vi "FormatTree&TableStyle.vi"(7 "Format Command":T1, 8 "Error In":errorcluster, 9 "Row Index":i32, 10 "Array of Table references":refnum<vi>[](array[refnum]), 11 "Array of Tree references":refnum<vi>[](array[refnum])) -> (0 "Error Out":errorcluster)   [LabVIEW 2012]
doc: "SciScan 1.2 160622\nThis VI implements the formatting of table data which includes highlighting, unhighlighting, and modifying visible rows (due to scrolling).\n\n<b>INPUTS</b>\n--------\n<b>Format Command </b> - Formatting action needs to be be taken\n<b>Table references array </b>- Array containing references of the tables of interest\n<b>Row </b>- Row number that needs to be fromatted"
uses:
  FormatTree&TableStyle_Commands.ctl
  <vilib>/Utility/miscctls.llb/LVRowAndColumnTypeDef.ctl
  <vilib>/Utility/miscctls.llb/LVNodeAndColumnTypeDef.ctl
  <vilib>/Utility/miscctls.llb/LVRowAndColumnUnsignedTypeDef.ctl
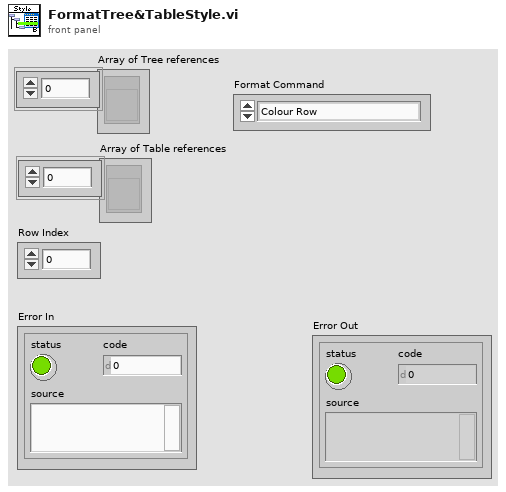
[diagram p1: front panel]
types:
  T1 = typedef "FormatTree&TableStyle_Commands.ctl" = enum16{"Colour Row", "Uncolour Row", "Bold Row", "Unbold Row", "Clear", "UpdateVisibleRows"}
  T2 = typedef "LVRowAndColumnTypeDef.ctl" = cluster{"Row":i32, "Column":i32}
  T3 = typedef "LVRowAndColumnUnsignedTypeDef.ctl" = cluster{"Row":u32, "Column":u32}
  T4 = typedef "LVNodeAndColumnTypeDef.ctl" = cluster{"Node":string, "Column":i32}
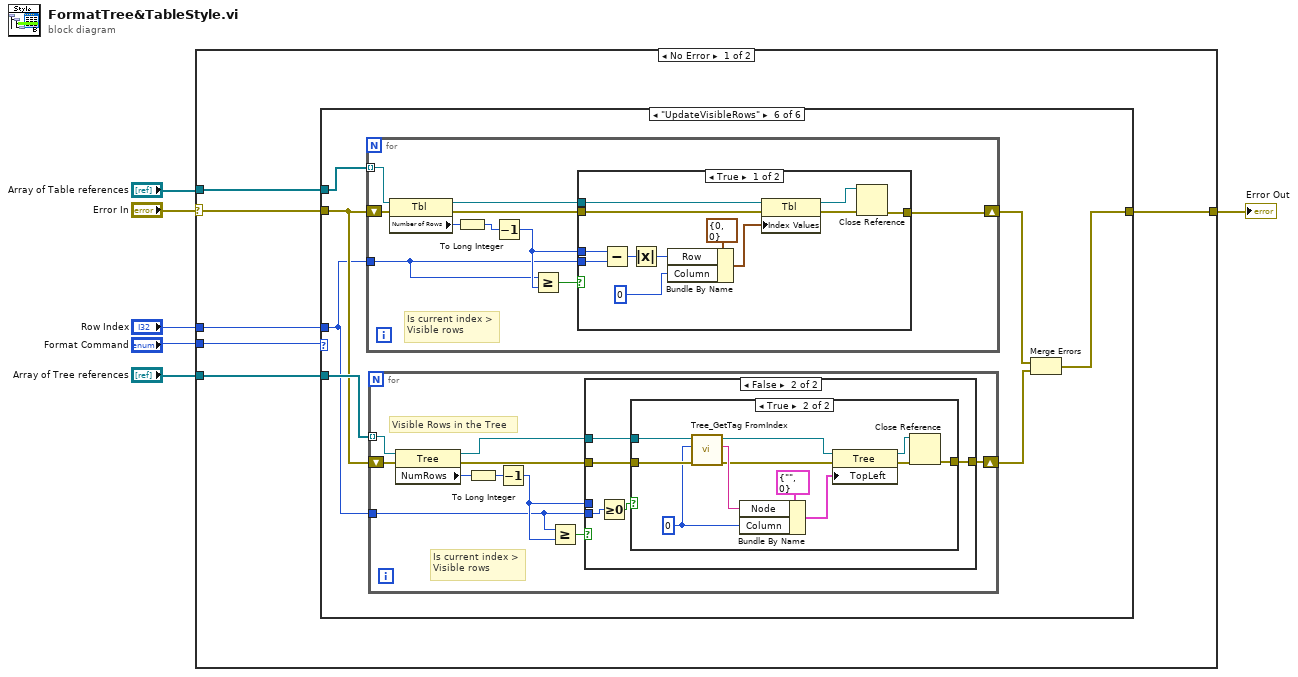
[diagram p0: block diagram]
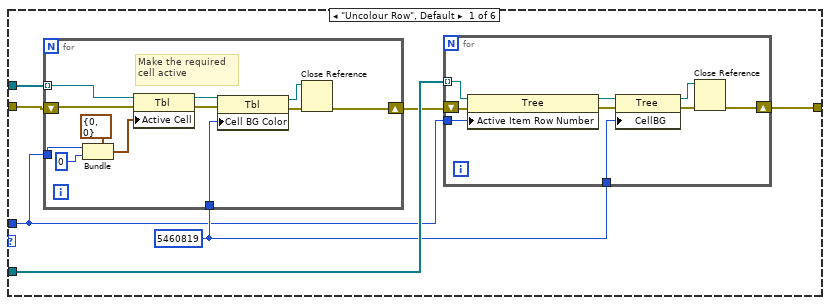
[diagram p2: hidden frame]
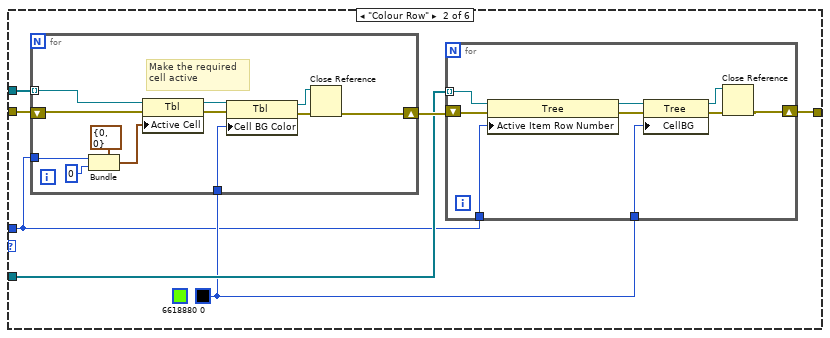
[diagram p3: hidden frame]
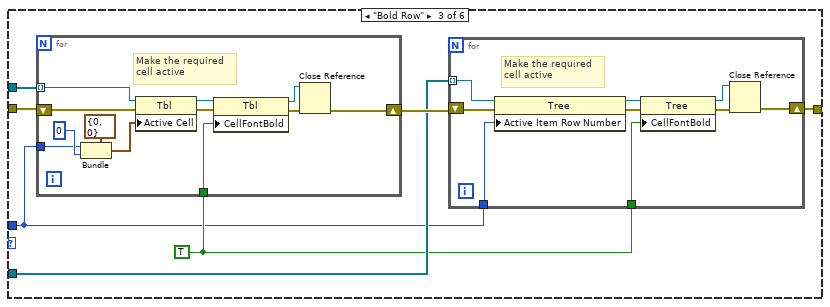
[diagram p4: hidden frame]
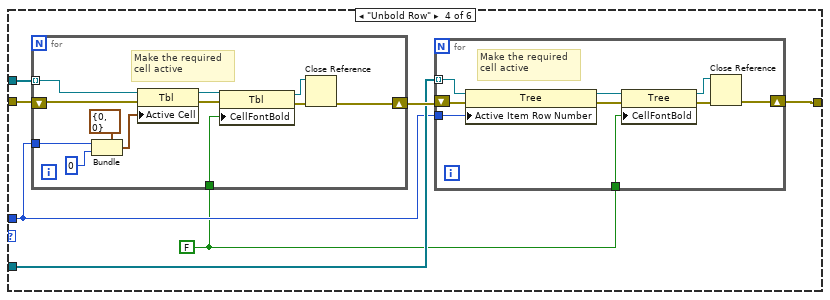
[diagram p5: hidden frame]
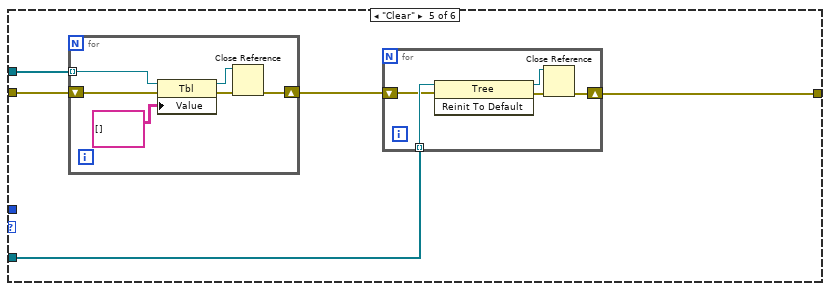
[diagram p6: hidden frame]
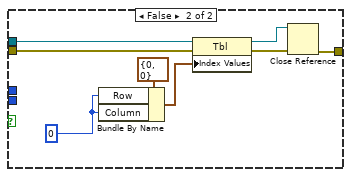
[diagram p7: hidden frame]
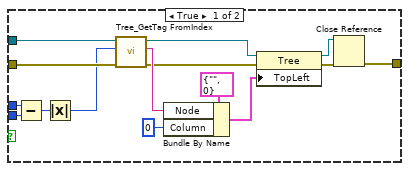
[diagram p8: hidden frame]
diagram:
  n1 = case shown="No Error" "Error In" {
    selector: "Error In" -> [w12 w220]
    tunnel: "Row Index" -> [w10 _]
    tunnel: [w9 w220] -> w4
    tunnel: "Array of Table references" -> [w11 _]
    tunnel: "Format Command" -> [w8 _]
    tunnel: "Array of Tree references" -> [w7 _]
    frame No Error {
      n2 = case shown="\"UpdateVisibleRows\"" w8 {
        tunnel: w12 -> [w19 w46 w74 w102 w128 w145]
        tunnel: w11 -> [w18 w45 w73 w101 w129 w146]
        tunnel: w10 -> [w13 w41 w69 w99 _ w144]
        tunnel: [w15 w43 w71 w98 w125 w141] -> w9
        tunnel: w7 -> [w17 w44 w72 w100 w127 w147]
        frame "Uncolour Row", Default {
          w14 = u32 5460819 ("Active Cell:Cell Background Color")
          n3 = for {
            tunnel: w18 -> [w26] mode=indexing
            tunnel: w14 -> [w24]
            shift-right: [w25] -> w16
            shift-left: w19 -> [w27]
            tunnel: w13 -> [w20]
            # "Make the required cell active"
            n4 = Bundle(cluster=T2 {"Row"=0, "Column"=0} ("Active Cell:Active Cell"), "Row"=w20, "Column"=0) -> (w22:T2)
            n5 = property class="Tbl"(reference=w26, error in=w27, "Active Cell"=w22) -> (reference out=w31:refnum<vi>, error out=w30:errorcluster)
            n6 = property class="Tbl"(reference=w31, error in=w30, "Cell BG Color"=w24) -> (reference out=w28:refnum<vi>, error out=w29:errorcluster)
            n7 = Close Reference(reference=w28, error in (no error)=w29) -> (error out=w25:errorcluster)
          }
          n8 = for {
            tunnel: w17 -> [w40] mode=indexing
            tunnel: w13 -> [w39]
            tunnel: w14 -> [w32]
            shift-right: [w33] -> w15
            shift-left: w16 -> [w36]
            n9 = property class="Tree"(reference=w40, error in=w36, "Active Item Row Number"=w39) -> (reference out=w37:refnum<vi>, error out=w38:errorcluster)
            n10 = property class="Tree"(reference=w37, error in=w38, "CellBG"=w32) -> (reference out=w34:refnum<vi>, error out=w35:errorcluster)
            n11 = Close Reference(reference=w34, error in (no error)=w35) -> (error out=w33:errorcluster)
          }
        }
        frame "Colour Row" {
          w42 = u32 0 ("Background colour")
          (unwired) u32 6618880 ("Background colour")
          n12 = for {
            tunnel: w45 -> [w53] mode=indexing
            tunnel: w42 -> [w52]
            shift-right: [w55] -> w47
            shift-left: w46 -> [w54]
            tunnel: w41 -> [w48]
            # "Make the required cell active"
            n13 = Bundle(cluster=T2 {"Row"=0, "Column"=0} ("Active Cell:Active Cell"), "Row"=w48, "Column"=0) -> (w49:T2)
            n14 = property class="Tbl"(reference=w53, error in=w54, "Active Cell"=w49) -> (reference out=w59:refnum<vi>, error out=w58:errorcluster)
            n15 = property class="Tbl"(reference=w59, error in=w58, "Cell BG Color"=w52) -> (reference out=w56:refnum<vi>, error out=w57:errorcluster)
            n16 = Close Reference(reference=w56, error in (no error)=w57) -> (error out=w55:errorcluster)
          }
          n17 = for {
            tunnel: w44 -> [w63] mode=indexing
            tunnel: w41 -> [w62]
            tunnel: w42 -> [w60]
            shift-right: [w61] -> w43
            shift-left: w47 -> [w66]
            n18 = property class="Tree"(reference=w63, error in=w66, "Active Item Row Number"=w62) -> (reference out=w67:refnum<vi>, error out=w68:errorcluster)
            n19 = property class="Tree"(reference=w67, error in=w68, "CellBG"=w60) -> (reference out=w64:refnum<vi>, error out=w65:errorcluster)
            n20 = Close Reference(reference=w64, error in (no error)=w65) -> (error out=w61:errorcluster)
          }
        }
        frame "Bold Row" {
          w70 = TRUE ("Active Cell:Cell Font:Bold")
          n21 = for {
            tunnel: w73 -> [w81] mode=indexing
            tunnel: w70 -> [w80]
            shift-right: [w83] -> w75
            shift-left: w74 -> [w82]
            tunnel: w69 -> [w77]
            # "Make the required cell active"
            n22 = Bundle(cluster=T2 {"Row"=0, "Column"=0} ("Active Cell:Active Cell"), "Row"=w77, "Column"=0) -> (w76:T2)
            n23 = property class="Tbl"(reference=w81, error in=w82, "Active Cell"=w76) -> (reference out=w87:refnum<vi>, error out=w86:errorcluster)
            n24 = property class="Tbl"(reference=w87, error in=w86, "CellFontBold"=w80) -> (reference out=w84:refnum<vi>, error out=w85:errorcluster)
            n25 = Close Reference(reference=w84, error in (no error)=w85) -> (error out=w83:errorcluster)
          }
          n26 = for {
            tunnel: w72 -> [w91] mode=indexing
            tunnel: w69 -> [w90]
            tunnel: w70 -> [w88]
            shift-right: [w89] -> w71
            shift-left: w75 -> [w94]
            # "Make the required cell active"
            n27 = property class="Tree"(reference=w91, error in=w94, "Active Item Row Number"=w90) -> (reference out=w95:refnum<vi>, error out=w96:errorcluster)
            n28 = property class="Tree"(reference=w95, error in=w96, "CellFontBold"=w88) -> (reference out=w92:refnum<vi>, error out=w93:errorcluster)
            n29 = Close Reference(reference=w92, error in (no error)=w93) -> (error out=w89:errorcluster)
          }
        }
        frame "Unbold Row" {
          w97 = FALSE ("Active Cell:Cell Font:Bold")
          n30 = for {
            tunnel: w101 -> [w106] mode=indexing
            tunnel: w99 -> [w105]
            tunnel: w97 -> [w104]
            shift-right: [w108] -> w103
            shift-left: w102 -> [w107]
            # "Make the required cell active"
            n31 = Bundle(cluster=T2 {"Row"=0, "Column"=0} ("Active Cell:Active Cell"), "Row"=w105, "Column"=0) -> (w110:T2)
            n32 = property class="Tbl"(reference=w106, error in=w107, "Active Cell"=w110) -> (reference out=w115:refnum<vi>, error out=w114:errorcluster)
            n33 = property class="Tbl"(reference=w115, error in=w114, "CellFontBold"=w104) -> (reference out=w112:refnum<vi>, error out=w113:errorcluster)
            n34 = Close Reference(reference=w112, error in (no error)=w113) -> (error out=w108:errorcluster)
          }
          n35 = for {
            tunnel: w100 -> [w119] mode=indexing
            tunnel: w99 -> [w118]
            tunnel: w97 -> [w116]
            shift-right: [w117] -> w98
            shift-left: w103 -> [w122]
            # "Make the required cell active"
            n36 = property class="Tree"(reference=w119, error in=w122, "Active Item Row Number"=w118) -> (reference out=w123:refnum<vi>, error out=w124:errorcluster)
            n37 = property class="Tree"(reference=w123, error in=w124, "CellFontBold"=w116) -> (reference out=w120:refnum<vi>, error out=w121:errorcluster)
            n38 = Close Reference(reference=w120, error in (no error)=w121) -> (error out=w117:errorcluster)
          }
        }
        frame "Clear" {
          n39 = for {
            tunnel: w129 -> [w135] mode=indexing
            shift-right: [w130] -> w126
            shift-left: w128 -> [w134]
            n40 = property class="Tbl"(reference=w135, error in=w134, "Value"=string[][] []) -> (reference out=w131:refnum<vi>, error out=w133:errorcluster)
            n41 = Close Reference(reference=w131, error in (no error)=w133) -> (error out=w130:errorcluster)
          }
          n42 = for {
            tunnel: w127 -> [w140] mode=indexing
            shift-right: [w136] -> w125
            shift-left: w126 -> [w139]
            n43 = invoke class="Tree" method="Reinit To Default"(reference=w140, error in=w139) -> (reference out=w137:refnum<vi>, error out=w138:errorcluster)  [unwired: 1 in, 1 out]
            n44 = Close Reference(reference=w137, error in (no error)=w138) -> (error out=w136:errorcluster)
          }
        }
        frame "UpdateVisibleRows" {
          n45 = for {
            tunnel: w146 -> [w154] mode=indexing
            shift-right: [w157] -> w143
            shift-left: w145 -> [w155]
            tunnel: w144 -> [w148]
            # "Is current index >\nVisible rows"
            n46 = property class="Tbl"(reference=w154, error in=w155) -> (reference out=w152:refnum<vi>, error out=w151:errorcluster, "Number of Rows"=w156:u32)
            n47 = To Long Integer(number=w156) -> (32bit integer=w150:i32)
            n48 = Decrement(x=w150) -> (x-1=w149:i32)
            n49 = Greater Or Equal?(x=w148, y=w149) -> (x >= y?=w153:bool)
            n50 = case shown="True" w153 {
              tunnel: [w169 w177] -> w157
              tunnel: w149 -> [w168 _]
              tunnel: w148 -> [w167 _]
              tunnel: w152 -> [w159 w172]
              tunnel: w151 -> [w158 w171]
              frame True {
                n51 = Subtract(x=w168, y=w167) -> (x-y=w161:i32)
                n52 = Absolute Value(x=w161) -> (abs(x)=w160:i32)
                n53 = Bundle By Name(cluster=T3 {"Row"=0, "Column"=0} ("Index Values"), "Row"=w160, "Column"=u32 0) -> (w162:T3)
                n54 = property class="Tbl"(reference=w159, error in=w158, "Index Values"=w162) -> (reference out=w164:refnum<vi>, error out=w165:errorcluster)
                n55 = Close Reference(reference=w164, error in (no error)=w165) -> (error out=w169:errorcluster)
              }
              frame False {
                w170 = u32 0 ("Column")
                n56 = Bundle By Name(cluster=T3 {"Row"=0, "Column"=0} ("Index Values"), "Row"=w170, "Column"=w170) -> (w173:T3)
                n57 = property class="Tbl"(reference=w172, error in=w171, "Index Values"=w173) -> (reference out=w174:refnum<vi>, error out=w175:errorcluster)
                n58 = Close Reference(reference=w174, error in (no error)=w175) -> (error out=w177:errorcluster)
              }
            }
          }
          n59 = for {
            tunnel: w144 -> [w178]
            tunnel: w147 -> [w184] mode=indexing
            shift-right: [w182] -> w142
            shift-left: w145 -> [w183]
            # "Is current index >\nVisible rows"
            # "Visible Rows in the Tree"
            n60 = property class="Tree"(reference=w184, error in=w183) -> (reference out=w186:refnum<vi>, error out=w187:errorcluster, "NumRows"=w185:u32)
            n61 = To Long Integer(number=w185) -> (32bit integer=w180:i32)
            n62 = Decrement(x=w180) -> (x-1=w179:i32)
            n63 = Greater Or Equal?(x=w178, y=w179) -> (x >= y?=w181:bool)
            n64 = case shown="False" w181 {
              tunnel: w187 -> [w202 w207]
              tunnel: w186 -> [w201 w206]
              tunnel: w179 -> [w200 _]
              tunnel: w178 -> [w199 w203]
              tunnel: [w197 w205] -> w182
              frame True {
                n65 = Subtract(x=w200, y=w199) -> (x-y=w196:i32)
                n66 = Absolute Value(x=w196) -> (abs(x)=w198:i32)
                n67 = call "Tree_GetTag FromIndex.vi"("Error In"=w202, "Index IN"=w198, "Tree Refnum IN"=w201) -> ("Error Out"=w191:errorcluster, "Tag OUT"=w193:string, "Tree Refnum OUT"=w192:refnum<vi>)  [unwired: 6 in]
                n68 = Bundle By Name(cluster=T4 {"Node"="", "Column"=0} ("Top Left Visible Cell"), "Node"=w193, "Column"=0) -> (w190:T4)
                n69 = property class="Tree"(reference=w192, error in=w191, "TopLeft"=w190) -> (reference out=w188:refnum<vi>, error out=w189:errorcluster)
                n70 = Close Reference(reference=w188, error in (no error)=w189) -> (error out=w197:errorcluster)
              }
              frame False {
                n71 = Greater Or Equal To 0?(x=w203) -> (x >= 0?=w204:bool)
                n72 = case shown="True" w204 {
                  tunnel: w207 -> [w208 w219]
                  tunnel: w206 -> [_ w218]
                  tunnel: [w208 w217] -> w205
                  frame False {
                  }
                  frame True {
                    w209 = 0 ("Column")
                    n73 = call "Tree_GetTag FromIndex.vi"("Error In"=w219, "Index IN"=w209, "Tree Refnum IN"=w218) -> ("Error Out"=w213:errorcluster, "Tag OUT"=w215:string, "Tree Refnum OUT"=w214:refnum<vi>)  [unwired: 6 in]
                    n74 = Bundle By Name(cluster=T4 {"Node"="", "Column"=0} ("Top Left Visible Cell"), "Node"=w215, "Column"=w209) -> (w212:T4)
                    n75 = property class="Tree"(reference=w214, error in=w213, "TopLeft"=w212) -> (reference out=w210:refnum<vi>, error out=w211:errorcluster)
                    n76 = Close Reference(reference=w210, error in (no error)=w211) -> (error out=w217:errorcluster)
                  }
                }
              }
            }
          }
          n77 = Merge Errors(w143, w142) -> (w141:errorcluster)
        }
      }
    }
    frame Error {
    }
  }
  "Error Out" <- w4
